vi "CLSUIP_InitVIRetooler.vi"(8 "error in (no error)":errorcluster, 9 "Replacement class":refnum<vi>, 10 "Member VI":refnum<vi>, 11 "VIRetooler in":refnum<class "VIRetooler.lvclass">) -> (0 "error out":errorcluster, 3 "VIRetooler out":refnum<class "VIRetooler.lvclass">)   [LabVIEW 2021, in "MemberVICreation.lvlib" / "VIRetooler.lvclass"]
uses:
  <resource>/Framework/Providers/LVClassLibrary/NewAccessors/VIRetooler/VIRetooler.lvclass
  <resource>/Framework/Providers/LVClassLibrary/NewAccessors/VIRetooler/VIRetooler.lvclass/VIRetooler.ctl
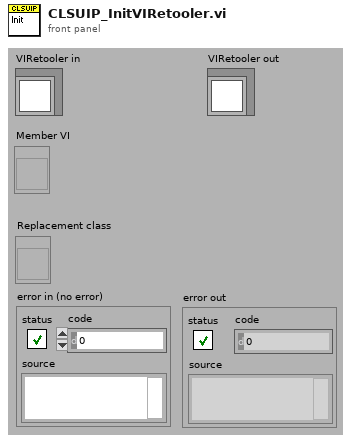
[diagram p1: front panel]
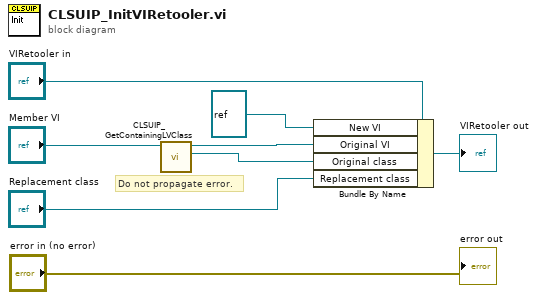
[diagram p0: block diagram]
diagram:
  # "Do not propagate error."
  n1 = call <resource>:"CLSUIP_GetContainingLVClass.vi"("Member VI"="Member VI") -> ("Containing LVClass"=w2:refnum<vi>, "Member VI out"=w1:refnum<vi>)  [unwired: 1 in, 8 out]
  n2 = Bundle By Name(cluster="VIRetooler in", "New VI"=refnum<vi> refnum, "Original VI"=w1, "Original class"=w2, "Replacement class"="Replacement class") -> (→"VIRetooler out":refnum<class "VIRetooler.lvclass">)
  "error out" <- "error in (no error)"
